vi "oa_Get Tach Points and Orbit Data from Resampled Data.vi"(0 "resampled signal in":cluster{"r0":dbl, "dr":dbl, "Y":dbl[]}[](array[cluster]) {"r0" format="%.2p"; "dr" format="%.2p"; "Y" format="%.2f"}, 1 "tach duty":i32=1, 11 "error in":errorcluster, 12 "trigger pulse direction":u16(ring)=1 items=["positive going", "negative going"]) -> (4 "tach points":cluster{dbl[], dbl[]} {"?" format="%.2f"; "?" format="%.2f"}, 6 "orbit":cluster{dbl[], dbl[]} {"?" format="%.2f"; "?" format="%.2f"}, 15 "error out":errorcluster)   [LabVIEW 2017]
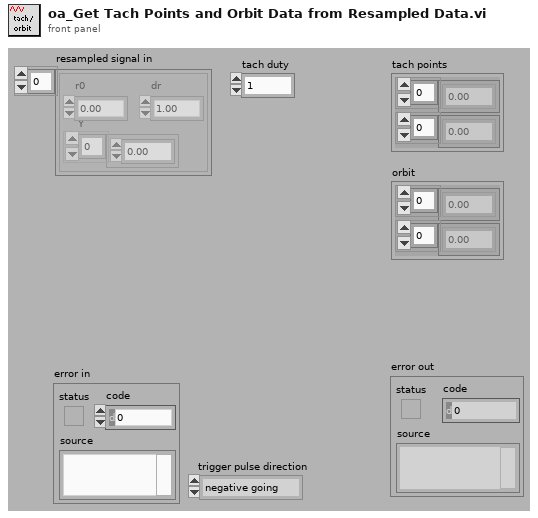
[diagram p1: front panel]
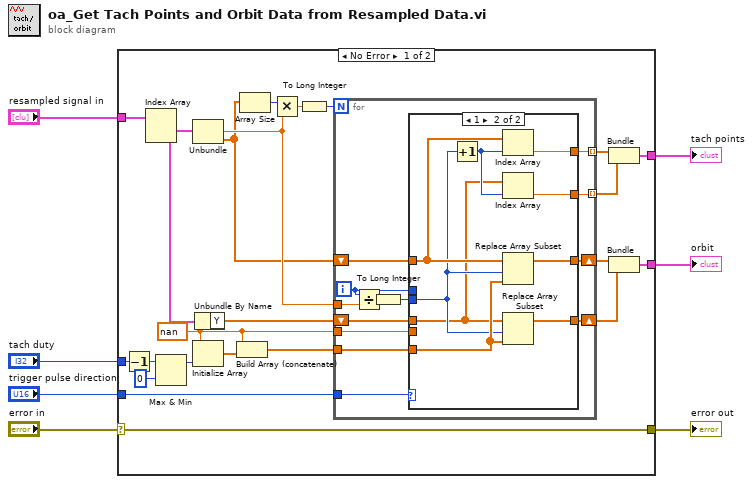
[diagram p0: block diagram]
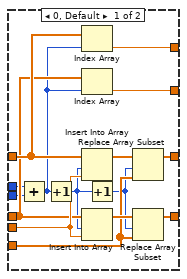
[diagram p2: hidden frame]
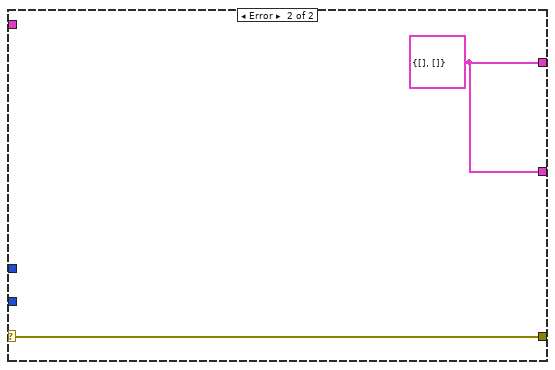
[diagram p3: hidden frame]
diagram:
  n1 = case shown="No Error" "error in" {
    selector: "error in" -> [w28 w70]
    tunnel: [w28 w70] -> w6
    tunnel: "resampled signal in" -> [w31 _]
    tunnel: [w21 w69] -> w3
    tunnel: [w25 w69] -> w4
    tunnel: "tach duty" -> [w20 _]
    tunnel: "trigger pulse direction" -> [w12 _]
    frame No Error {
      w15 = nan ("element")
      n2 = Decrement(x=w20) -> (x-1=w19:i32)
      n3 = Index Array(array=w31) -> (element #1=w30:cluster{"r0":dbl, "dr":dbl, "Y":dbl[]}, element #2=w29:cluster{"r0":dbl, "dr":dbl, "Y":dbl[]})  [unwired: 2 in]
      n4 = Max & Min(x=w19, y=0) -> (max(x,y)=w17:i32)  [unwired: 1 out]
      n5 = Unbundle(w30) -> ("dr"=w13:dbl, "Y"=w11:dbl[])  [unwired: 1 out]
      n6 = Initialize Array(w15, w17) -> (w16:dbl[])
      n7 = Unbundle By Name(w29) -> ("Y"=w10:dbl[])
      n8 = Build Array (concatenate)(w15, w16) -> (w14:dbl[])
      n9 = Array Size(array=w11) -> (size(s)=w27:i32)
      n10 = Multiply(x=w27, y=w13) -> (x*y=w26:dbl)
      n11 = To Long Integer(number=w26) -> (32bit integer=w24:i32)
      n12 = for {
        N: w24 -> [_]
        shift-right: [w43] -> w23
        shift-left: w11 -> [w44]
        shift-right: [w41] -> w22
        shift-left: w10 -> [w42]
        tunnel: w12 -> [w40]
        tunnel: w15 -> [w39]
        tunnel: w14 -> [w38]
        tunnel: w13 -> [w37]
        tunnel: [w34] -> w9 mode=indexing
        tunnel: [w33] -> w8 mode=indexing
        i -> [w36]
        n13 = Divide(x=w36, y=w37) -> (x/y=w35:dbl)
        n14 = To Long Integer(number=w35) -> (32bit integer=w32:i32)
        n15 = case shown="1" w40 {
          tunnel: w44 -> [w51 w66]
          tunnel: [w57 w68] -> w43
          tunnel: w42 -> [w49 w60]
          tunnel: w32 -> [w47 w61]
          tunnel: [w55 w67] -> w41
          tunnel: w39 -> [w59 _]
          tunnel: w38 -> [w54 w65]
          tunnel: w36 -> [w48 _]
          tunnel: [w52 w64] -> w34
          tunnel: [w50 w63] -> w33
          frame 0, Default {
            n16 = Add(x=w48, y=w47) -> (x+y=w46:i32)
            n17 = Increment(x=w46) -> (x+1=w45:i32)
            n18 = Index Array(array=w51, index=w46) -> (element=w52:dbl)
            n19 = Index Array(array=w49, index=w46) -> (element=w50:dbl)
            n20 = Insert Into Array(array=w51, index=w45, new element=w59) -> (w58:dbl[])
            n21 = Insert Into Array(array=w49, index=w45, new element=w59) -> (w56:dbl[])
            n22 = Increment(x=w45) -> (x+1=w53:i32)
            n23 = Replace Array Subset(array=w58, new element=w54, index=w53) -> (w57:dbl[])
            n24 = Replace Array Subset(array=w56, new element=w54, index=w53) -> (w55:dbl[])
          }
          frame 1 {
            n25 = Increment(x=w61) -> (x+1=w62:i32)
            n26 = Index Array(array=w66, index=w62) -> (element=w64:dbl)
            n27 = Index Array(array=w60, index=w62) -> (element=w63:dbl)
            n28 = Replace Array Subset(array=w66, new element=w65, index=w61) -> (w68:dbl[])
            n29 = Replace Array Subset(array=w60, new element=w65, index=w61) -> (w67:dbl[])
          }
        }
      }
      n30 = Bundle(w9, w8) -> (w25:cluster{dbl[], dbl[]})  [unwired: 1 in]
      n31 = Bundle("Y"=w23, "Y"=w22) -> (w21:cluster{"Y":dbl[], "Y":dbl[]})  [unwired: 1 in]
    }
    frame Error {
      w69 = cluster{dbl[], dbl[]} {[], []}
    }
  }
  "error out" <- w6
  "tach points" <- w4
  "orbit" <- w3
